vi "test3.vi"   [LabVIEW 2019]
uses:
  AK TCP/AK TCP.lvclass
  Protocol Parent/Protocol Parent.lvclass
  TCP/TCP.lvclass
  TCP/Data Access/Read Port.vi
  TCP/Data Access/Read TCP Ref.vi
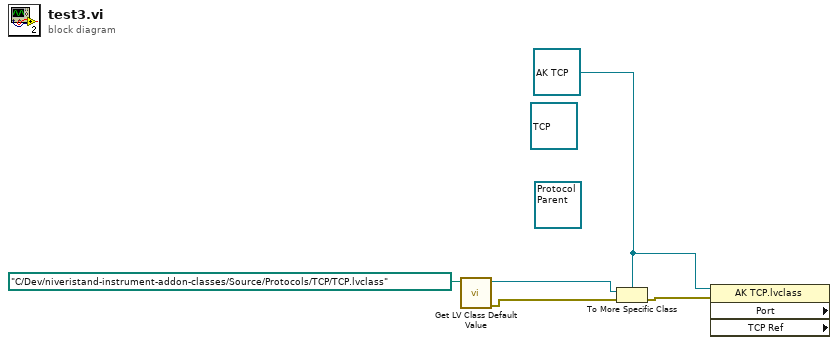
[diagram p0: block diagram]
diagram:
  w1 = refnum<class "AK TCP.lvclass"> refnum ("Protocols.lvlib:AK TCP.lvclass")
  (unwired) refnum<class "TCP.lvclass"> refnum ("Protocols.lvlib:TCP.lvclass")
  (unwired) refnum<class "Protocol Parent.lvclass"> refnum ("Protocols.lvlib:Protocol Parent.lvclass")
  n1 = call <vilib>:"Get LV Class Default Value.vi"("class path"=path "C:/Dev/niveristand-instrument-addon-classes/Source/Protocols/TCP/TCP.lvclass") -> ("error out"=w3:errorcluster, "object"=w4:refnum<class>)  [unwired: 9 in]
  n2 = To More Specific Class(target class=w1, reference=w4, error in=w3) -> (error out=w2:errorcluster)  [unwired: 1 out]
  n3 = property class="AK TCP.lvclass" props=["Port", "TCP Ref"](reference=w1, error in=w2) -> ()  [unwired: 4 out]
